vi "StellarNet Set Parameters.vi"(8 "error in":errorcluster, 11 "Settings":T1={"Integration Time (ms)"=80, "Temp  Compensation "=FALSE, "Optical Smoothing Level"=0, "Number of Scans to Average"=1, "Digitizer Clock Rate Setting"=3} {"Digitizer Clock Rate Setting" min=1 max=3; "Number of Scans to Average" min=1 max=10000 step=1; "Optical Smoothing Level" min=0 max=4 step=1}) -> (0 "error out":errorcluster)   [LabVIEW 2020, in "StellarNetSpectrometer.lvclass"]
doc: "Phisically send the spectrometer configuration to the device"
uses:
  StellarNetSpectrometer.lvclass
  Swdll.dll
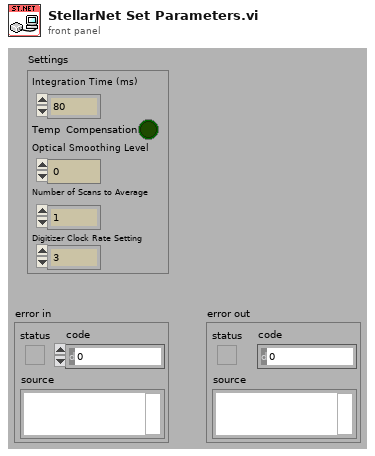
[diagram p1: front panel]
types:
  T1 = cluster{"Integration Time (ms)":i32, "Temp  Compensation ":bool, "Optical Smoothing Level":i32, "Number of Scans to Average":i32, "Digitizer Clock Rate Setting":i32}
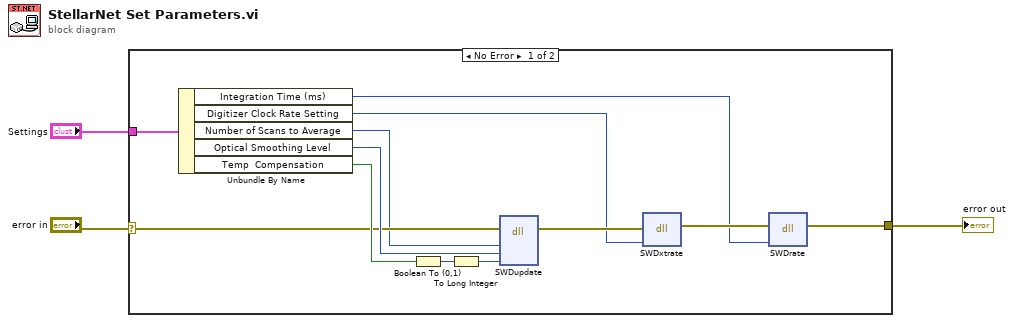
[diagram p0: block diagram]
diagram:
  n1 = case shown="No Error" "error in" {
    selector: "error in" -> [w6 w16]
    tunnel: [w15 w16] -> w3
    tunnel: "Settings" -> [w5 _]
    frame No Error {
      n2 = Unbundle By Name(w5) -> ("Integration Time (ms)"=w10:i32, "Digitizer Clock Rate Setting"=w9:i32, "Number of Scans to Average"=w4:i32, "Optical Smoothing Level"=w8:i32, "Temp  Compensation"=w7:bool)
      n3 = Boolean To (0,1)(Boolean=w7) -> (0, 1=w12:i16)
      n4 = To Long Integer(number=w12) -> (32bit integer=w13:i32)
      n5 = dll-call lib="C:/GEECS/Developers Version/source/Device Drivers/StellarNet Black-Comet Spec/SupportLib/StellarNetSpectrometerClass/CommMethods/Swdll.dll" fn="SWDupdate"(error in=w6, "ScansTo Avg"=w4, "Xsmooth"=w8, "TempComp"=w13) -> (error out=w11:errorcluster)  [unwired: 6 in, 1 out]
      n6 = dll-call lib="C:/GEECS/Developers Version/source/Device Drivers/StellarNet Black-Comet Spec/SupportLib/StellarNetSpectrometerClass/CommMethods/Swdll.dll" fn="SWDxtrate" label="xtrate"(error in=w11, "xtrate"=w9) -> (error out=w14:errorcluster)  [unwired: 4 in, 1 out]
      n7 = dll-call lib="C:/GEECS/Developers Version/source/Device Drivers/StellarNet Black-Comet Spec/SupportLib/StellarNetSpectrometerClass/CommMethods/Swdll.dll" fn="SWDrate"(error in=w14, "dsf"=w10) -> (error out=w15:errorcluster)  [unwired: 4 in, 1 out]
    }
    frame Error {
    }
  }
  "error out" <- w3
